vi "Default Settings.vi"(8 "error in (no error)":errorcluster, 11 "C4 Dispense in 2":refnum<class "Iterative Dispense.lvclass">) -> (0 "error out":errorcluster, 3 "C4 Dispense out 2":refnum<class "Iterative Dispense.lvclass">)   [LabVIEW 2020, in "Iterative Dispense.lvclass"]
uses:
  Iterative Dispense.lvclass
  Dispense.lvclass
panel:
  # "This Routine does not Accept Settings"
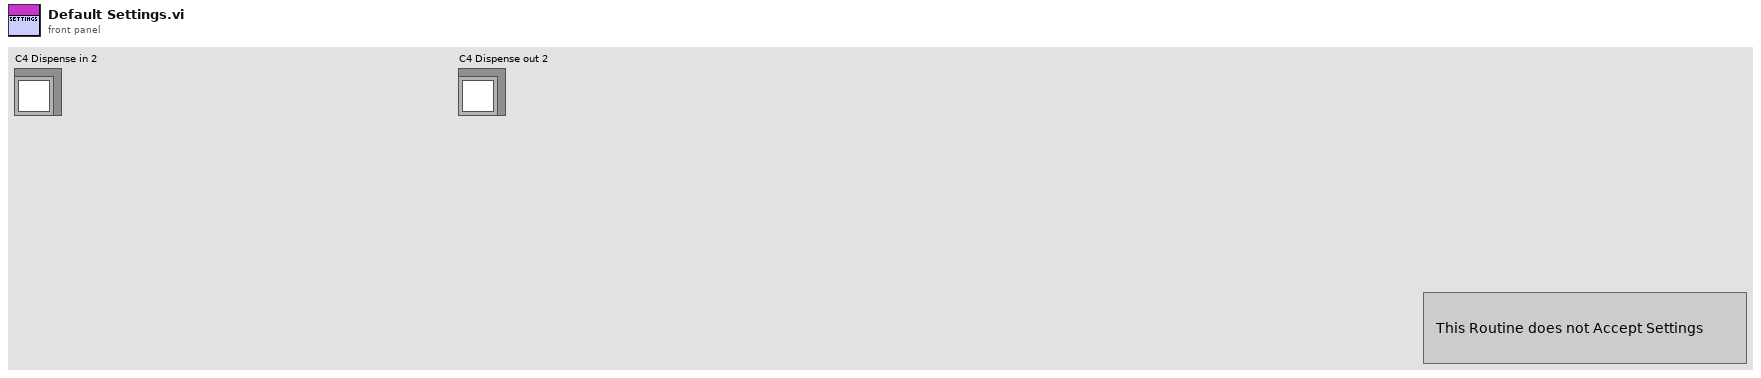
[diagram p1: front panel]
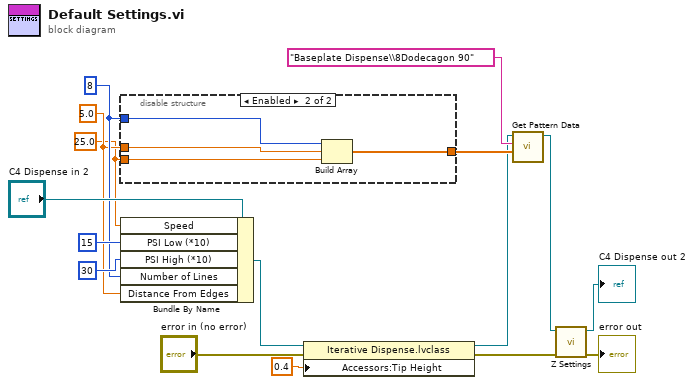
[diagram p0: block diagram]
diagram:
  w10 = 5.0 ("Edge Distance")
  w11 = 8 ("Lines")
  w9 = 25.0 ("Speed")
  n1 = disable-structure shown="Enabled" {
    disable-tunnel: w11 -> [_ w20]
    disable-tunnel: w10 -> [_ w19]
    disable-tunnel: w9 -> [_ w18]
    disable-tunnel: [_ w17] -> w8
    frame Disabled {
    }
    frame Enabled {
      n2 = Build Array(w20, w19, w18) -> (w17:dbl[])
    }
  }
  n3 = Bundle By Name(cluster="C4 Dispense in 2", "Speed"=w9, "PSI Low (*10)"=15, "PSI High (*10)"=30, "Number of Lines"=w11, "Distance From Edges"=w10) -> (w6:refnum<class "Iterative Dispense.lvclass">)
  n4 = property class="Iterative Dispense.lvclass"(reference=w6, error in="error in (no error)", "Accessors:Tip Height"=0.4 ("Tip Height")) -> (reference out=w5:refnum<class "Iterative Dispense.lvclass">, error out=w2:errorcluster)
  n5 = call "Get Pattern Data.vi"("File Name"=w8, "Folder Name"="Baseplate Dispense\\8Dodecagon 90", "Dispense.lvclass"=w5) -> ("Dispense Out"=w4:refnum<class "Iterative Dispense.lvclass">)  [unwired: 8 in]
  n6 = call-dynamic "Z Settings.vi"("error in (no error)"=w2, "Dispense in"=w4) -> ("error out"=→"error out":errorcluster, "Dispense out"=→"C4 Dispense out 2":refnum<class "Iterative Dispense.lvclass">)  [unwired: 8 in]
